vi "GetFileRefNum.vi"(8 "Error IN":errorcluster caption="에러 입력", 10 "FilePath":path, 11 "HEKAdat.lvclass IN":refnum<class "HEKAdat.lvclass">) -> (0 "Error OUT":errorcluster caption="에러 출력", 2 "FilePath":path, 3 "HEKAdat.lvclass OUT":refnum<class "HEKAdat.lvclass">)   [LabVIEW 2017, in "HEKAdat.lvclass"]
uses:
  HEKAdat.lvclass
  HEKAdat.lvclass/HEKAdat.ctl
panel:
  out "size (in bytes)":i64
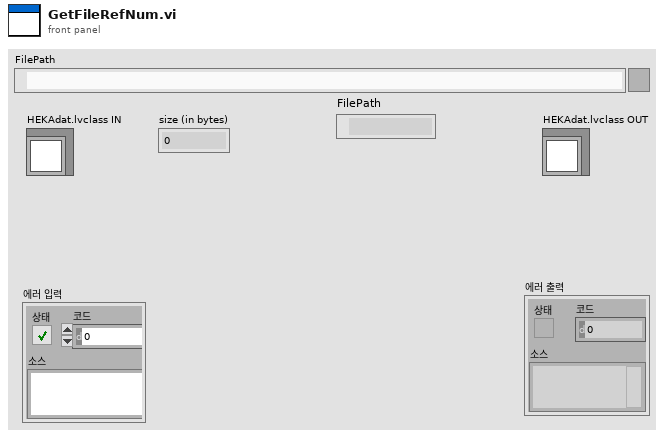
[diagram p1: front panel]
types:
  T1 = enum16{"open", "replace", "create", "open or create", "replace or create", "replace or create with confirmation"}
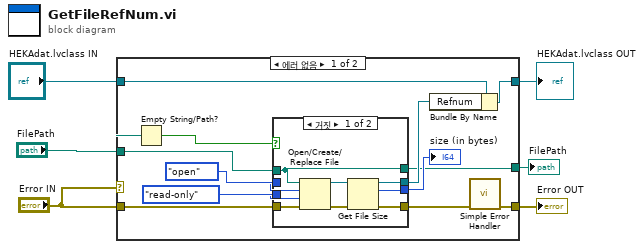
[diagram p0: block diagram]
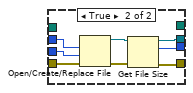
[diagram p2: hidden frame]
diagram:
  n1 = case shown="에러 없음" "Error IN" {
    tunnel: "Error IN" -> [w18 w36]
    tunnel: [w17 w36] -> w6
    tunnel: "HEKAdat.lvclass IN" -> [w11 w37]
    tunnel: [w10 w37] -> w4
    tunnel: "FilePath" -> [w15 _]
    tunnel: [w7 _] -> w1
    frame No Error {
      n2 = Empty String/Path?(string/path=w15) -> (empty?=w16:bool)
      n3 = case shown="거짓" w16 {
        tunnel: w18 -> [w25 w33]
        tunnel: w15 -> [w19 _]
        tunnel: T1."open" ("operation (0:open)") -> [w27 w35]
        tunnel: enum16{"read/write", "read-only", "write-only"}."read-only" ("access (0:read/write)") -> [w26 w34]
        tunnel: [w21 w29] -> w12
        tunnel: [w23 w31] -> w9
        tunnel: [w20 w28] -> w8
        tunnel: [w19 _] -> w7
        frame False {
          n4 = Open/Create/Replace File(file path (use dialog)=w19, error in=w25, operation (0:open)=w27, access (0:read/write)=w26) -> (refnum out=w24:refnum<file>, error out=w22:errorcluster)  [unwired: 2 in, 1 out]
          n5 = Get File Size(file=w24, error in=w22) -> (refnum out=w23:refnum<file>, size (in bytes)=w20:i64, 0:w21:errorcluster)
        }
        frame True {
          n6 = Open/Create/Replace File(error in=w33, operation (0:open)=w35, access (0:read/write)=w34) -> (refnum out=w32:refnum<file>, error out=w30:errorcluster)  [unwired: 3 in, 1 out]
          n7 = Get File Size(file=w32, error in=w30) -> (refnum out=w31:refnum<file>, size (in bytes)=w28:i64, 0:w29:errorcluster)
        }
      }
      "size (in bytes)" <- w8
      n8 = Bundle By Name(cluster=w11, "Refnum"=w9) -> (w10:refnum<class "HEKAdat.lvclass">)
      n9 = call <vilib>:"Simple Error Handler.vi"("error in (no error)"=w12) -> ("error out"=w17:errorcluster)  [unwired: 4 in, 4 out]
    }
    frame Error {
    }
  }
  "Error OUT" <- w6
  "HEKAdat.lvclass OUT" <- w4
  "FilePath" <- w1
